vi "EvaluateNode.vi"(8 "error in (no error)":errorcluster, 10 "ToEvaluate in":refnum<data-value>, 11 "Tree in":refnum<class "Tree.lvclass">) -> (0 "error out":errorcluster, 2 "ToEvaluate out":refnum<data-value>, 3 "Tree out":refnum<class "Tree.lvclass">)   [LabVIEW 2014, in "Tree.lvlib" / "Tree.lvclass"]
doc: "Evaluates a node and sets the to ToSortBy value. This is used to determine the position the node should go into Open."
uses:
  <userlib>/AdvancedDataStructures/ClassBased/Tree/Tree.lvclass
  <userlib>/AdvancedDataStructures/ClassBased/TreeNode/TreeNode.lvclass
  <userlib>/AdvancedDataStructures/ClassBased/Common/BasicSortedList/BasicSortedNode/BasicSortedNode.lvclass
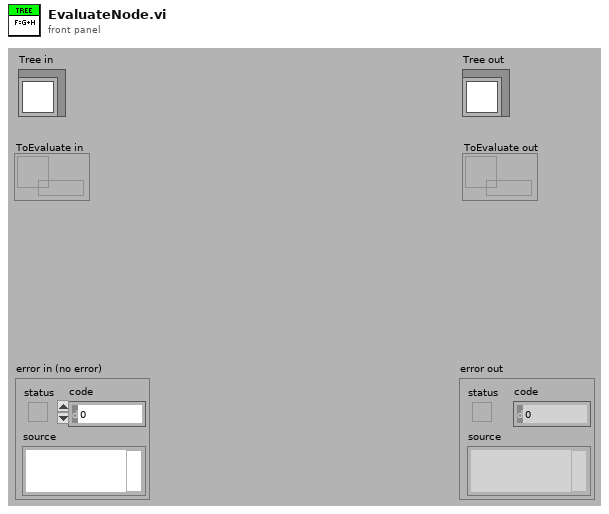
[diagram p1: front panel]
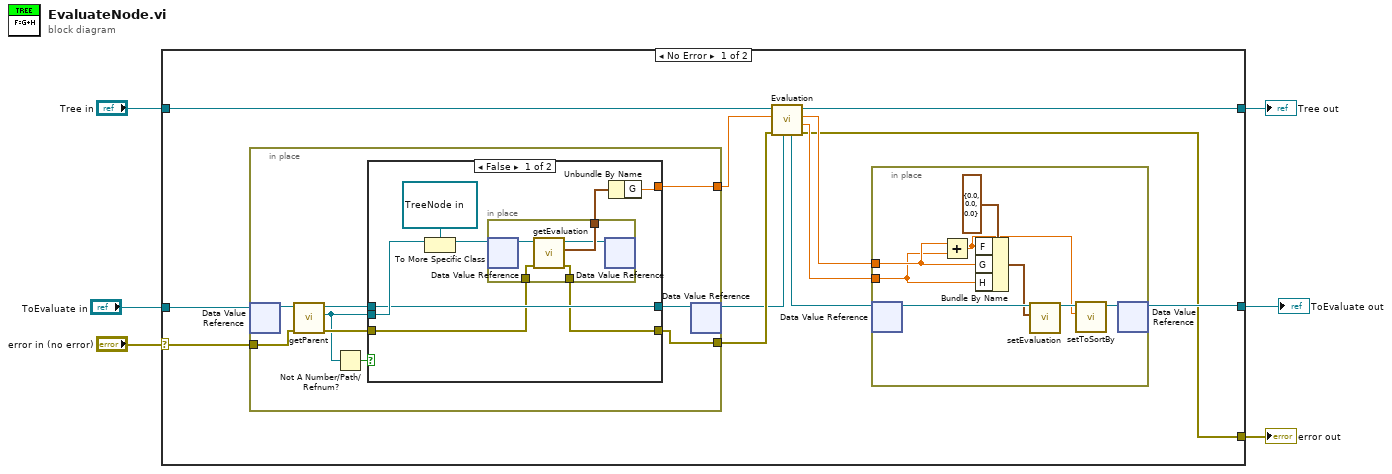
[diagram p0: block diagram]
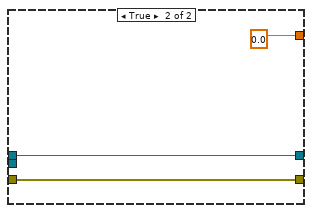
[diagram p2: hidden frame]
diagram:
  n1 = case shown="No Error" "error in (no error)" {
    selector: "error in (no error)" -> [w17 w54]
    tunnel: [w7 w54] -> w5
    tunnel: [w15 w53] -> w3
    tunnel: "Tree in" -> [w16 w53]
    tunnel: "ToEvaluate in" -> [w18 w52]
    tunnel: [w10 w52] -> w1
    frame No Error {
      n2 = in-place {
        in-place-border: w17 -> [w29]
        in-place-border: [w28] -> w14
        in-place-border: [w27] -> w13
        n3 = in-place-dvr #1(w18) -> (w31:refnum<class "TreeNode.lvclass">)  [unwired: 1 out]
        n4 = call <userlib>:"getParent.vi"("error in (no error)"=w29, "TreeNode in"=w31) -> ("error out"=w34:errorcluster, "Parent"=w32:refnum<data-value>, "TreeNode out"=w33:refnum<class "TreeNode.lvclass">)  [unwired: 7 in]
        n5 = Not A Number/Path/Refnum?(number/path/refnum=w32) -> (NaN/Path/Refnum?=w35:bool)
        n6 = case shown="False" w35 {
          tunnel: w34 -> [w39 w50]
          tunnel: w33 -> [w41 w51]
          tunnel: w32 -> [w43 _]
          tunnel: [w41 w51] -> w30
          tunnel: [w38 w50] -> w28
          tunnel: [w36 0.0 ("Parents G")] -> w27
          frame False {
            n7 = To More Specific Class(target class=refnum<data-value> refnum ("data value reference"), reference=w43) -> (specific class reference=w40:refnum<data-value>)  [unwired: 1 in, 1 out]
            n8 = in-place {
              in-place-border: w39 -> [w47]
              in-place-border: [w46] -> w38
              in-place-border: [w45] -> w37
              n9 = in-place-dvr #2(w40) -> (w48:refnum<class "TreeNode.lvclass">)  [unwired: 1 out]
              n10 = call <userlib>:"getEvaluation.vi"("error in (no error)"=w47, "TreeNode in"=w48) -> ("error out"=w46:errorcluster, "evaluation"=w45:cluster{"F":dbl, "G":dbl, "H":dbl}, "TreeNode out"=w44:refnum<class "TreeNode.lvclass">)  [unwired: 7 in]
              n11 = in-place-dvr #2(w44) -> ()  [unwired: 2 out]
            }
            n12 = Unbundle By Name(w37) -> ("G"=w36:dbl)
          }
          frame True {
          }
        }
        n13 = in-place-dvr #1(w30) -> (w12:refnum<data-value>)  [unwired: 1 out]
      }
      n14 = call-dynamic "Evaluation.vi"("ToEvaluate in"=w12, "error in (no error)"=w14, "Parents G"=w13, "Tree in"=w16) -> ("error out"=w7:errorcluster, "H"=w8:dbl, "G"=w9:dbl, "Tree out"=w15:refnum<class "Tree.lvclass">, "ToEvaluate out"=w11:refnum<data-value>)  [unwired: 3 in]
      n15 = in-place {
        in-place-border: w9 -> [w24]
        in-place-border: w8 -> [w23]
        n16 = in-place-dvr #3(w11) -> (w26:refnum<class "TreeNode.lvclass">)  [unwired: 1 out]
        n17 = Add(x=w24, y=w23) -> (x+y=w19:dbl)
        n18 = Bundle By Name(cluster=cluster{"F":dbl, "G":dbl, "H":dbl} {"F"=0.0, "G"=0.0, "H"=0.0} ("evaluation"), "F"=w19, "G"=w24, "H"=w23) -> (w22:cluster{"F":dbl, "G":dbl, "H":dbl})
        n19 = call <userlib>:"setEvaluation.vi"("evaluation"=w22, "TreeNode in"=w26) -> ("TreeNode out"=w21:refnum<class "TreeNode.lvclass">)  [unwired: 8 in, 1 out]
        n20 = call <userlib>:"setToSortBy.vi"("ToSortBy"=w19, "BasicSortedNode in"=w21) -> ("BasicSortedNode out"=w20:refnum<class "TreeNode.lvclass">)  [unwired: 8 in, 1 out]
        n21 = in-place-dvr #3(w20) -> (w10:refnum<data-value>)  [unwired: 1 out]
      }
    }
    frame Error {
    }
  }
  "error out" <- w5
  "Tree out" <- w3
  "ToEvaluate out" <- w1
